vi "Run_1_of_X_Tests.vi"() -> ()   [LabVIEW 2019]
uses:
  <vilib>/Rock Robotics/WPI/ThirdParty/JAS_Junk/TrajLib/Trajectory_Library.lvlib
panel:
  out "Diff Drive Odom 2":bool
  out "String":string
  out "Diff Drive Kine Constraint":bool
  out "Diff Drive Voltage Constraint":bool
  out "Bang Bang Input/Output":bool
  out "Bang Bang Tolerance":bool
  out "All Tests Finished":bool
  out "Centrip Accel Constraint":bool
  out "Controller Utility":bool
  out "Chassis Speeds":bool
  out "Cubic Spline":bool
  out "Diff Drive Kinematics":bool
  out "Angle Stats":bool
  # "FORMAL TRAJECTORY / CONTROL LIBRARY TEST PROCEDURE"
  # "FUNCTION NOT\nIMPLEMENTED"
  # "Cntrl Affine Plant Inversion"
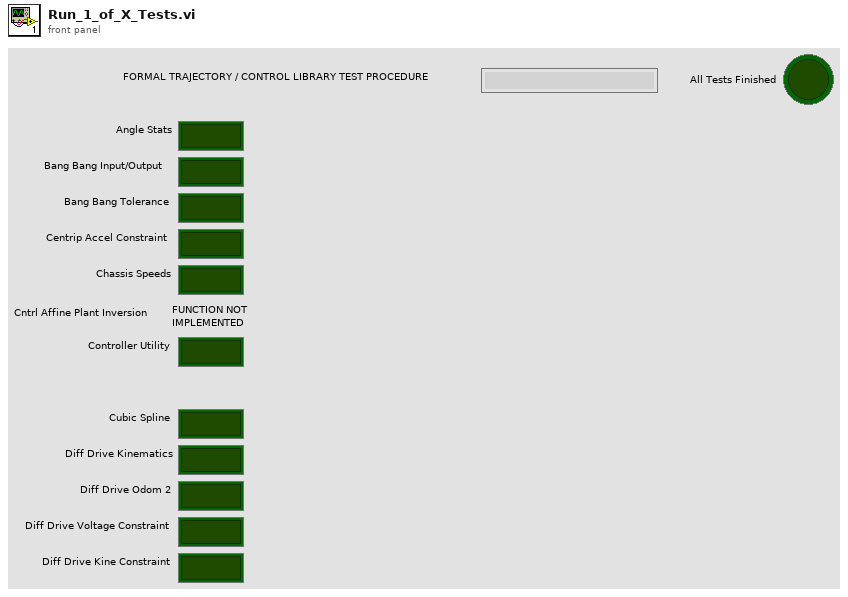
[diagram p1: front panel]
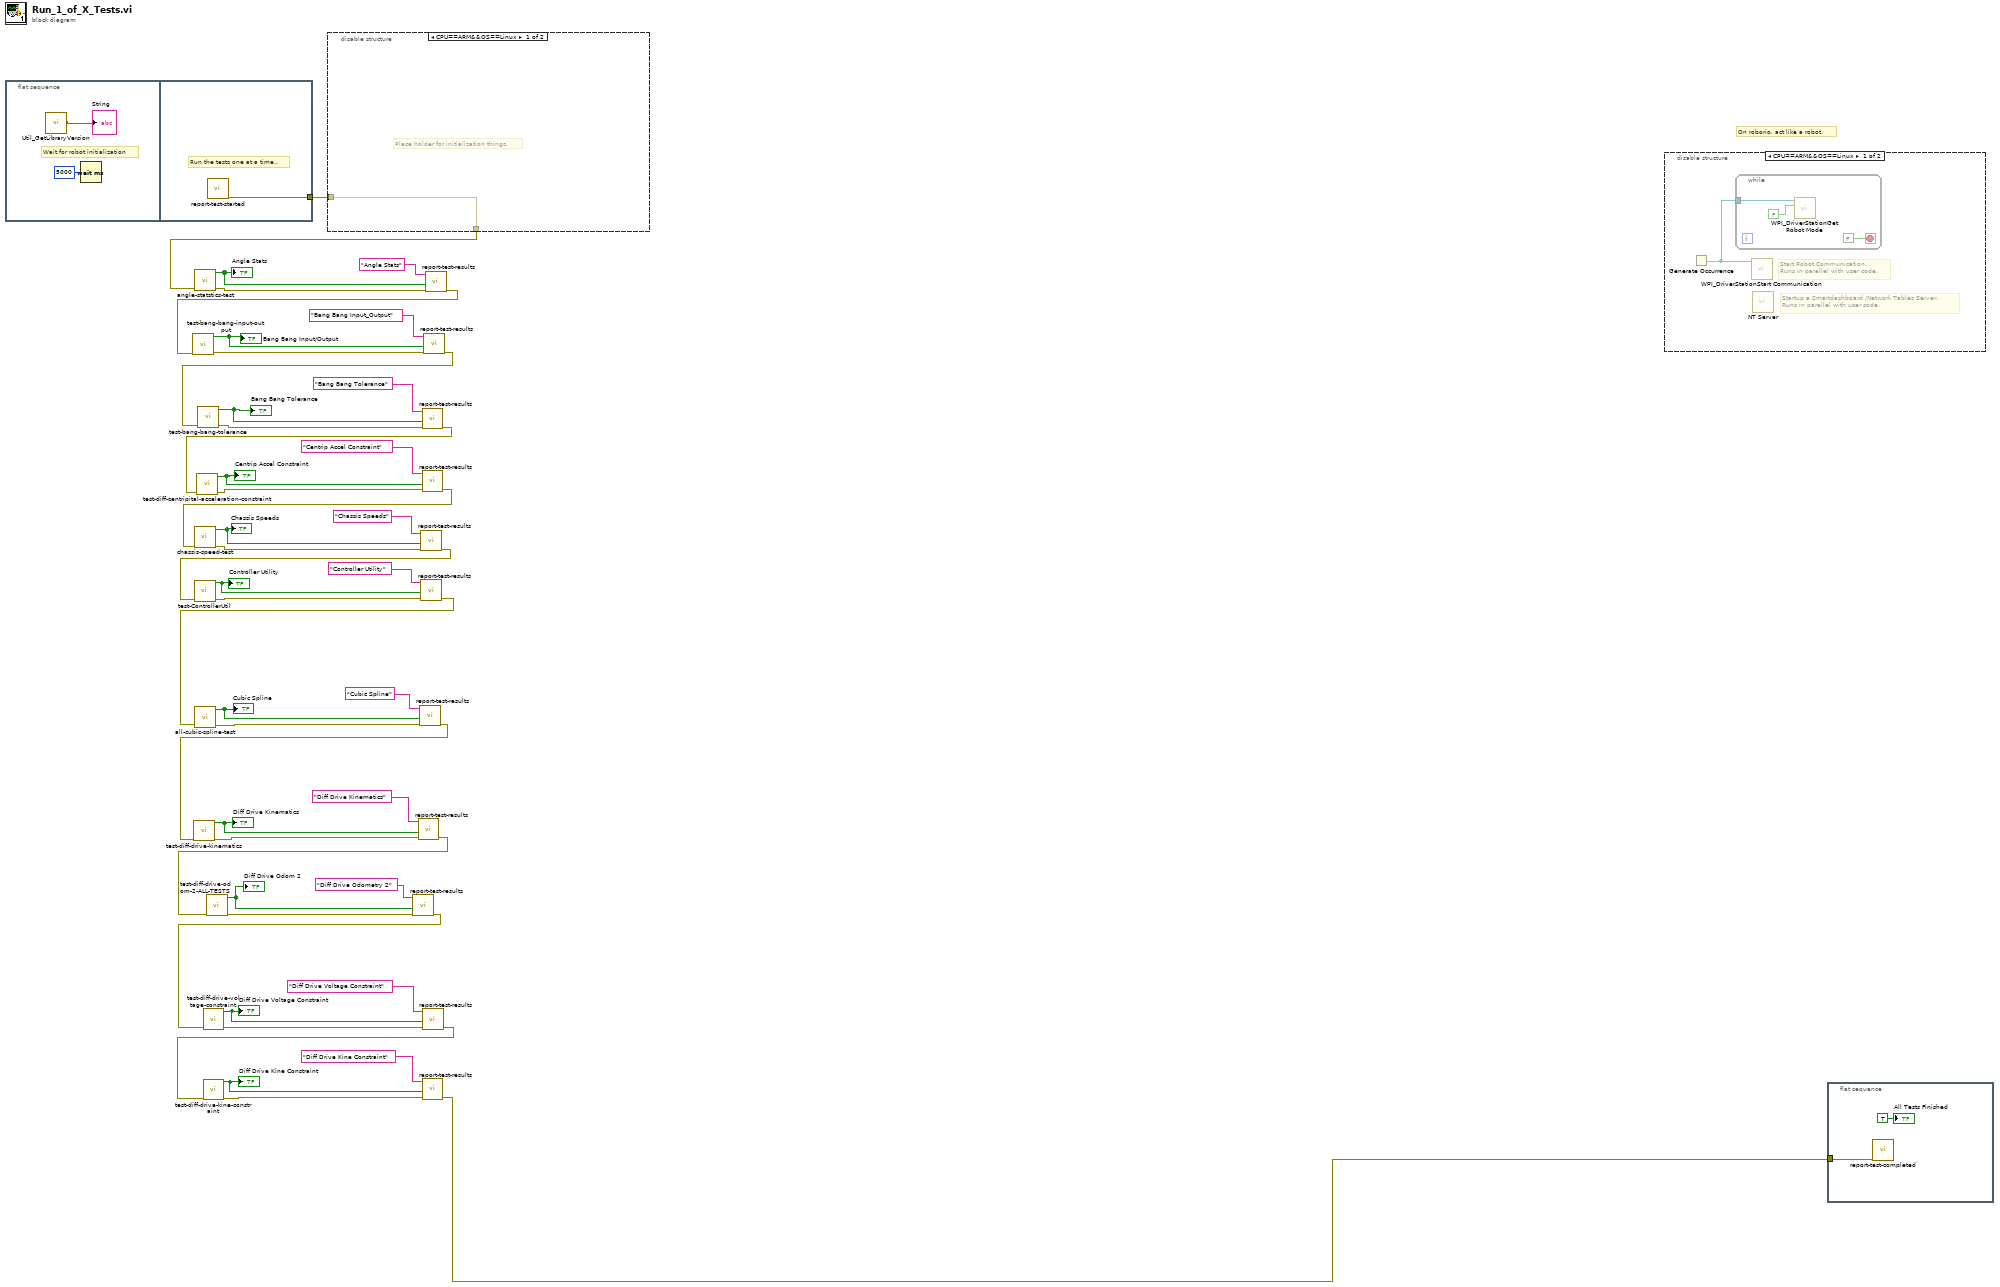
[diagram p0: block diagram]
diagram:
  # "On roborio, act like a robot."
  n1 = flat-sequence {
    tunnel: [w49] -> w17
    frame #0 {
      # "Wait for robot initialization"
      n2 = call <vilib>:"Util_GetLibraryVersion.vi"() -> ("TrajLibVersion"=→"String":string)  [unwired: 11 in]
      n3 = Wait (ms)(milliseconds to wait=u32 5000) -> ()  [unwired: 1 out]
    }
    frame #1 {
      # "Run the tests one at a time.."
      n4 = call "report-test-started.vi"() -> ("error out"=w49:errorcluster)  [unwired: 11 in]
    }
  }
  n5 = disable-structure shown="CPU==ARM&&OS==Linux" {
    disable-tunnel: w17 -> [w50 w51]
    disable-tunnel: [w50 w51] -> w16
    frame condition #0 {
      # "Place holder for initialization things."
    }
    frame condition #1 (active) {
    }
  }
  n6 = call "angle-statstics-test.vi"("error in (no error)"=w16) -> ("error out"=w30:errorcluster, "All Passed"=w46:bool)  [unwired: 9 in]
  "Angle Stats" <- w46
  n7 = call "report-test-results.vi"("error in (no error)"=w30, "TestPassed"=w46, "Test Name"="Angle Stats") -> ("error out"=w29:errorcluster)  [unwired: 8 in]
  n8 = call "test-bang-bang-input-output.vi"("error in (no error)"=w29) -> ("error out"=w28:errorcluster, "All Tests Passed"=w43:bool)  [unwired: 9 in]
  "Bang Bang Input/Output" <- w43
  n9 = call "report-test-results.vi"("error in (no error)"=w28, "TestPassed"=w43, "Test Name"="Bang Bang Input_Output") -> ("error out"=w27:errorcluster)  [unwired: 8 in]
  n10 = call "test-bang-bang-tolerance.vi"("error in (no error)"=w27) -> ("error out"=w26:errorcluster, "All Tests Passed"=w41:bool)  [unwired: 9 in]
  "Bang Bang Tolerance" <- w41
  n11 = call "report-test-results.vi"("error in (no error)"=w26, "TestPassed"=w41, "Test Name"="Bang Bang Tolerance") -> ("error out"=w25:errorcluster)  [unwired: 8 in]
  n12 = call "test-diff-centripital-acceleration-constraint.vi"("error in (no error)"=w25) -> ("error out 2"=w24:errorcluster, "Test Passed"=w39:bool)  [unwired: 9 in]
  "Centrip Accel Constraint" <- w39
  n13 = call "report-test-results.vi"("error in (no error)"=w24, "TestPassed"=w39, "Test Name"="Centrip Accel Constraint") -> ("error out"=w23:errorcluster)  [unwired: 8 in]
  n14 = call "chassis-speed-test.vi"("error in (no error)"=w23) -> ("error out"=w22:errorcluster, "Test Passed"=w37:bool)  [unwired: 9 in]
  "Chassis Speeds" <- w37
  n15 = call "report-test-results.vi"("error in (no error)"=w22, "TestPassed"=w37, "Test Name"="Chassis Speeds") -> ("error out"=w21:errorcluster)  [unwired: 8 in]
  n16 = call "test-ControllerUtil.vi"("error in (no error)"=w21) -> ("error out"=w20:errorcluster, "All Tests Passed"=w35:bool)  [unwired: 9 in]
  "Controller Utility" <- w35
  n17 = call "report-test-results.vi"("error in (no error)"=w20, "TestPassed"=w35, "Test Name"="Controller Utility") -> ("error out"=w6:errorcluster)  [unwired: 8 in]
  n18 = call "all-cubic-spline-test.vi"("error in (no error)"=w6) -> ("error out"=w19:errorcluster, "ALL TESTS PASSED"=w32:bool)  [unwired: 9 in]
  "Cubic Spline" <- w32
  n19 = call "report-test-results.vi"("error in (no error)"=w19, "TestPassed"=w32, "Test Name"="Cubic Spline") -> ("error out"=w7:errorcluster)  [unwired: 8 in]
  n20 = call "test-diff-drive-kinematics.vi"("error in (no error)"=w7) -> ("error out"=w18:errorcluster, "All Passed"=w31:bool)  [unwired: 9 in]
  "Diff Drive Kinematics" <- w31
  n21 = call "report-test-results.vi"("error in (no error)"=w18, "TestPassed"=w31, "Test Name"="Diff Drive Kinematics") -> ("error out"=w2:errorcluster)  [unwired: 8 in]
  n22 = call "test-diff-drive-odom-2-ALL-TESTS.vi"("error in (no error)"=w2) -> ("error out"=w4:errorcluster, "All Passed"=w3:bool)  [unwired: 9 in]
  "Diff Drive Odom 2" <- w3
  n23 = call "report-test-results.vi"("error in (no error)"=w4, "TestPassed"=w3, "Test Name"="Diff Drive Odometry 2") -> ("error out"=w1:errorcluster)  [unwired: 8 in]
  n24 = call "test-diff-drive-voltage-constraint.vi"("error in (no error)"=w1) -> ("error out 4"=w13:errorcluster, "Test Passed"=w14:bool)  [unwired: 9 in]
  "Diff Drive Voltage Constraint" <- w14
  n25 = call "report-test-results.vi"("error in (no error)"=w13, "TestPassed"=w14, "Test Name"="Diff Drive Voltage Constraint") -> ("error out"=w9:errorcluster)  [unwired: 8 in]
  n26 = call "test-diff-drive-kine-constraint.vi"("error in (no error)"=w9) -> ("error out 2"=w10:errorcluster, "Test Passed"=w11:bool)  [unwired: 9 in]
  "Diff Drive Kine Constraint" <- w11
  n27 = call "report-test-results.vi"("error in (no error)"=w10, "TestPassed"=w11, "Test Name"="Diff Drive Kine Constraint") -> ("error out"=w8:errorcluster)  [unwired: 8 in]
  n28 = disable-structure shown="CPU==ARM&&OS==Linux" {
    frame condition #0 {
      # "Startup a Smartdashboard /Network Tables Server.\nRuns in parallel with user code."
      # "Start Robot Communication.\nRuns in parallel with user code."
      n29 = Generate Occurrence() -> (w52:refnum<k4>)
      n30 = while {
        tunnel: w52 -> [w55]
        stop <- FALSE stop-if-true
        n31 = call <vilib>:"WPI_DriverStationGet Robot Mode.vi"("Finish"=FALSE, "DS Occurrence"=w55) -> ()  [unwired: 10 out]
      }
      n32 = call <vilib>:"WPI_DriverStationStart Communication.vi"("occurrence"=w52) -> ()  [unwired: 2 in, 9 out]
      n33 = call <vilib>:"NT Server.vi"() -> ()  [unwired: 12 in]
    }
    frame condition #1 (active) {
    }
  }
  n34 = flat-sequence {
    tunnel: w8 -> [w56]
    frame #0 {
      n35 = call "report-test-completed.vi"("error in (no error)"=w56) -> ()  [unwired: 10 in, 1 out]
      "All Tests Finished" <- TRUE ("All Tests Finished")
    }
  }
